vi "SetStrikeout.vi"(8 "error in (no error)":errorcluster, 10 "Strikeout?":bool, 11 "Font in":refnum<class "Font.lvclass">) -> (0 "error out":errorcluster, 3 "Font out":refnum<class "Font.lvclass">)   [LabVIEW 2021, in "Picture2D.lvlib" / "Font.lvclass"]
uses:
  Font.lvclass
  Font.lvclass/Font.ctl
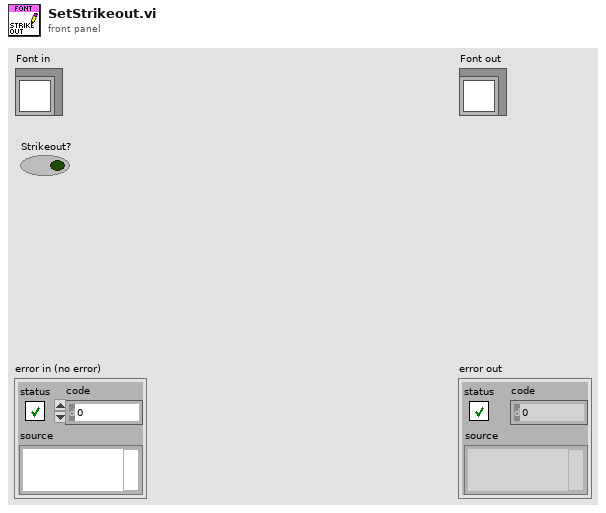
[diagram p1: front panel]
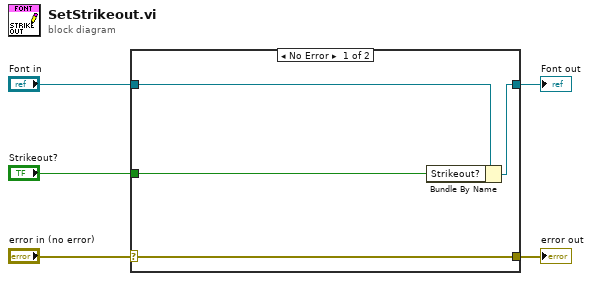
[diagram p0: block diagram]
diagram:
  n1 = case shown="No Error" "error in (no error)" {
    selector: "error in (no error)" -> [w9 w10]
    tunnel: [w9 w10] -> w4
    tunnel: [w7 w11] -> w2
    tunnel: "Font in" -> [w8 w11]
    tunnel: "Strikeout?" -> [w6 _]
    frame No Error {
      n2 = Bundle By Name(cluster=w8, "Strikeout?"=w6) -> (w7:refnum<class "Font.lvclass">)
    }
    frame Error {
    }
  }
  "error out" <- w4
  "Font out" <- w2
